vi "CheckIfGObjectMatches.vi"(8 "error in (no error)":errorcluster, 10 "GObj Refnum":refnum<vi>, 11 "XControl Layout in":refnum<class "XControl Layout.lvclass">) -> (0 "error out":errorcluster, 2 "compatible?":bool)   [LabVIEW 2010, in "NI_SE_Front Panel Layout.lvlib" / "XControl Layout.lvclass"]
uses:
  XControl Layout.lvclass
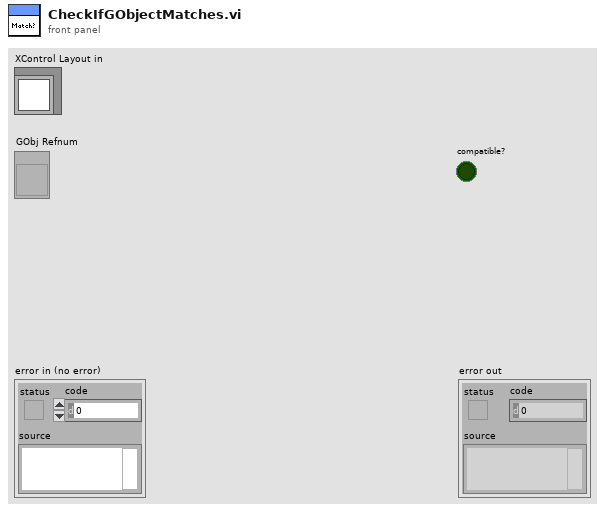
[diagram p1: front panel]
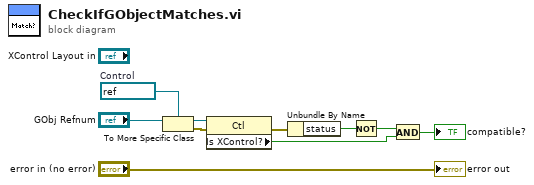
[diagram p0: block diagram]
diagram:
  w8 = refnum<vi> refnum  # Control
  n1 = To More Specific Class(target class=w8, reference="GObj Refnum") -> (specific class reference=w7:refnum<vi>, error out=w6:errorcluster)  [unwired: 1 in]
  n2 = property class="Ctl"(reference=w7, error in=w6) -> (error out=w5:errorcluster, "Is XControl?"=w3:bool)  [unwired: 1 out]
  n3 = Unbundle By Name(w5) -> ("status"=w1:bool)
  n4 = Not(x=w1) -> (.not. x?=w4:bool)
  n5 = And(x=w4, y=w3) -> (x .and. y?=→"compatible?":bool)
  "error out" <- "error in (no error)"
